vi "Gyro PID Fwd Color Stop.vi"(5 "Port":T1 items=["Port 1", "Port 2", "Port 3", "Port 4"], 6 "Target angle":sgl, 7 "Threshold to Color":i32=1200, 8 "Threshold to slow":i32=1000, 9 "Min. speed":i32=40, 10 "Max. speed":i32=80, 11 "EV3 in":T2) -> (3 "EV3 out":T2)   [LabVIEW 2016]
uses:
  <vilib>/NXT/Subs/LVHSConnector.ctl
  <vilib>/NXT/LegoClasses/BrickReference/BrickReference.lvclass
  <vilib>/NXT/Block Support/NXT_InputPort.ctl
  <vilib>/NXT/Block Support/NXT_OutputPort.ctl
  <vilib>/NXT/NXTIO Xnodes/NXTIONodeSubVIs/LEGOResetMotors.vi
  <vilib>/NXT/Dual Mode Library/Motors/Rotation.vi
  <vilib>/NXT/Dual Mode Library/Sensors/EV3_Color_Reflect.vi
  <vilib>/NXT/NXTIO Xnodes/NXTIONodeSubVIs/NXTMotorSteeringOn.vi
  <vilib>/NXT/NXTIO Xnodes/NXTIONodeSubVIs/NXTStopMotors.vi
  <vilib>/NXT/Dual Mode Library/Waits/Wait_Num.vi
  <vilib>/NXT/NXTIO Xnodes/NXTIOXNode/NXTIO.xnode
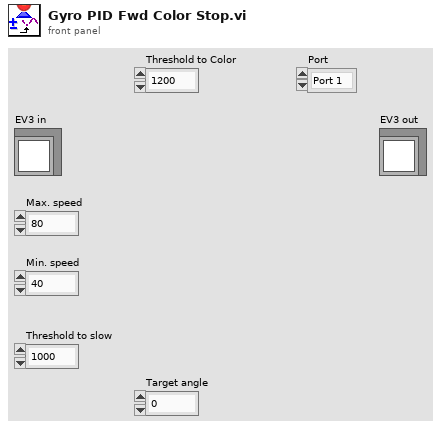
[diagram p1: front panel]
types:
  T1 = typedef "NXT_InputPort.ctl" = u32
  T2 = typedef "LVHSConnector.ctl" = refnum<class "BrickReference.lvclass">
  T3 = typedef "NXT_OutputPort.ctl" = u8
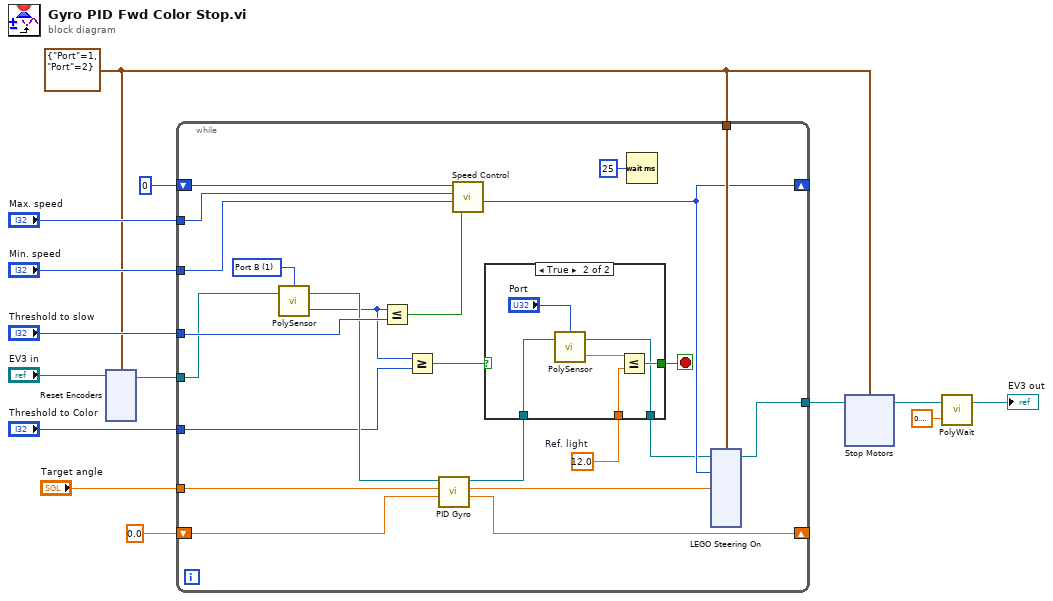
[diagram p0: block diagram]
diagram:
  w4 = cluster{"Port":T3, "Port":T3} {"Port"=1, "Port"=2} ("Motor")
  n1 = xnode "Reset Encoders"("Motors"=w4, "NXT/EV3"="EV3 in") -> ("NXT/EV3"=w10:T2)
  n2 = while {
    tunnel: w10 -> [w26]
    shift-right: [w37] -> _
    shift-left: sgl 0.0 -> [w22]
    tunnel: "Target angle" -> [w36]
    tunnel: [w33] -> w6
    tunnel: w4 -> [w35]
    shift-right: [w21] -> _
    shift-left: 0 -> [w30]
    tunnel: "Min. speed" -> [w27]
    tunnel: "Max. speed" -> [w29]
    tunnel: "Threshold to slow" -> [w28]
    tunnel: "Threshold to Color" -> [w20]
    stop <- w19 stop-if-true
    w15 = sgl 12.0  # Ref. light
    w34 = T3 1 items=["Port A", "Port B", "Port C", "Port D"] ("Port (Port A)")
    n3 = call-poly <vilib>:"PolySensor.vi"("NXT/EV3"=w26, "Port (Port A)"=w34) -> ("Angle of Rotation"=w23:i32, "NXT/EV3"=w25:T2)  [unwired: 1 in]
    n4 = Less Or Equal?(x=w23, y=w28) -> (x <= y?=w24:bool)
    n5 = Greater Or Equal?(x=w23, y=w20) -> (x >= y?=w18:bool)
    n6 = call "PID Gyro.vi"("Previous integral"=w22, "Target angle"=w36, "EV3 in"=w25) -> ("New integral"=w37:sgl, "Total error"=w31:sgl, "EV3 out"=w17:T2)  [unwired: 6 in]
    n7 = call "Speed Control.vi"("Speed Up or Down?"=w24, "Min. speed"=w27, "Max. speed"=w29, "Ini. speed"=w30) -> ("Speed out"=w21:i32)  [unwired: 7 in]
    n8 = case shown="True" w18 {
      tunnel: [_ w42] -> w19
      tunnel: w17 -> [w38 w41]
      tunnel: [w38 w40] -> w16
      tunnel: w15 -> [_ w39]
      frame False {
      }
      frame True {
        n9 = call-poly <vilib>:"PolySensor.vi"("NXT/EV3"=w41, "Port (Port 1)"="Port") -> ("Scaled Value"=w43:sgl, "NXT/EV3"=w40:T2)  [unwired: 1 in]
        n10 = Less Or Equal?(x=w43, y=w39) -> (x <= y?=w42:bool)
      }
    }
    n11 = Wait (ms)(milliseconds to wait=u32 25) -> ()  [unwired: 1 out]
    n12 = xnode "LEGO Steering On"("Steering 1"=w31, "Power 1"=w21, "Motors"=w35, "NXT/EV3"=w16) -> ("NXT/EV3"=w33:T2)
  }
  n13 = xnode "Stop Motors"("Motors"=w4, "NXT/EV3"=w6) -> ("NXT/EV3"=w5:T2)
  n14 = call-poly <vilib>:"PolyWait.vi"("Time (1 sec)"=sgl 0.2, "NXT/EV3"=w5) -> ("NXT/EV3"=→"EV3 out":T2)  [unwired: 2 in]
